vi "Move Knot.vi"(7 "Previous knot":cluster{"X":i32, "Y":i32}, 11 "Current Knot In":cluster{"X":i32, "Y":i32}) -> (3 "Current Knot Out":cluster{"X":i32, "Y":i32})   [LabVIEW 2021]
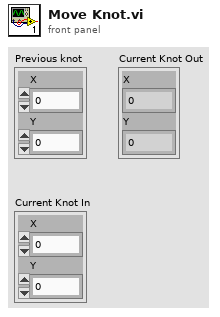
[diagram p1: front panel]
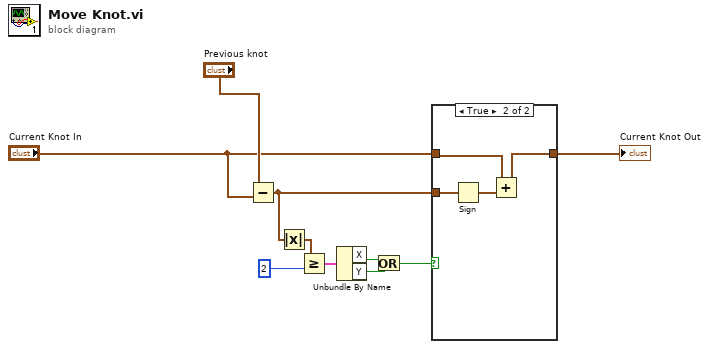
[diagram p0: block diagram]
diagram:
  n1 = Subtract(x="Previous knot", y="Current Knot In") -> (x-y=w8:cluster{"X":i32, "Y":i32})
  n2 = Absolute Value(x=w8) -> (abs(x)=w5:cluster{"X":i32, "Y":i32})
  n3 = Greater Or Equal?(x=w5, y=2) -> (x >= y?=w2:cluster{"X":bool, "Y":bool})
  n4 = Unbundle By Name(w2) -> ("X"=w3:bool, "Y"=w4:bool)
  n5 = Or(x=w3, y=w4) -> (x .or. y?=w6:bool)
  n6 = case shown="True" w6 {
    tunnel: "Current Knot In" -> [w11 w13]
    tunnel: [w11 w12] -> w10
    tunnel: w8 -> [_ w15]
    frame False {
    }
    frame True {
      n7 = Sign(1:w15) -> (0:w14:cluster{"X":i32, "Y":i32})
      n8 = Add(x=w13, y=w14) -> (x+y=w12:cluster{"X":i32, "Y":i32})
    }
  }
  "Current Knot Out" <- w10
